vi "UpdateLifecycle.vi"(10 "Lifecycle":T1, 11 "Actor":refnum<class "Actor.lvclass">) -> (3 "Actor":refnum<class "Actor.lvclass">)   [LabVIEW 2020, in "jettl.lvlib"]
uses:
  jettl.lvlib
  Actor/Actor.lvclass
  LifecycleEnum.ctl
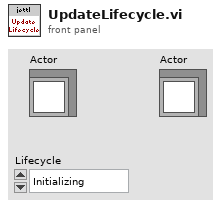
[diagram p1: front panel]
types:
  T1 = typedef "jettl.lvlib/LifecycleEnum.ctl" = enum16{"Initializing", "SettingUp", "Starting", "Running", "Stopping", "TearingDown", "Terminated"}
  T2 = typedef "jettl.lvlib/BaseCluster.ctl" = cluster{"LifecycleEnum":T1, "MainCluster":T3, "SelfActorCluster":T4, "MediatorActorCluster":T4, "ComponentActorClusterMap":T9}
  T3 = typedef "jettl.lvlib/MainCluster.ctl" = cluster{"PreSetupClusterQueue":refnum<queue>, "BeginSetupQueue":refnum<queue>, "SetupErrorQueue":refnum<queue>, "BeginStartQueue":refnum<queue>}
  T4 = typedef "jettl.lvlib/ActorCluster.ctl" = cluster{"MessagesCluster":T5, "Alias":string, "ActorType":T8, "Transport":refnum<user-event>, "EventRegistrationRef":refnum<event-registration>, "VIRef":refnum<vi>}
  T5 = typedef "jettl.lvlib/MessagesCluster.ctl" = cluster{"ListenMessageSet":T6, "TellSelfMessageSet":T6, "TellMediatorMessageSet":T6, "TellComponentMessageSetMap":T7}
  T6 = typedef "jettl.lvlib/MessageSet.ctl" = set{refnum<class "Message.lvclass">}
  T7 = typedef "jettl.lvlib/TellComponentMessageSetMap.ctl" = map{string, T6}
  T8 = typedef "jettl.lvlib/ActorTypeEnum.ctl" = enum16{"Mediator", "Component"}
  T9 = typedef "jettl.lvlib/ComponentActorClusterMap.ctl" = map{string, T4}
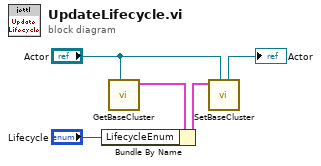
[diagram p0: block diagram]
diagram:
  n1 = call-dynamic "GetBaseCluster.vi"("Actor"="Actor") -> ("BaseCluster"=w5:T2)  [unwired: 10 in]
  n2 = Bundle By Name(cluster=w5, "LifecycleEnum"="Lifecycle") -> (w4:T2)
  n3 = call-dynamic "SetBaseCluster.vi"("Actor"="Actor", "BaseCluster"=w4) -> ("Actor"=→"Actor":refnum<class "Actor.lvclass">)  [unwired: 9 in]
